vi "_appendClusterFlattenedData.vi"(8 "error in (no error)":errorcluster, 10 "Variant Data":variant, 11 "Flattened Cluster":string) -> (0 "error out":errorcluster, 3 "Appended Cluster":string)   [LabVIEW 2013, in "BSON.lvlib" / "tBSONDocument.lvclass"]
uses:
  tBSONDocument.lvclass
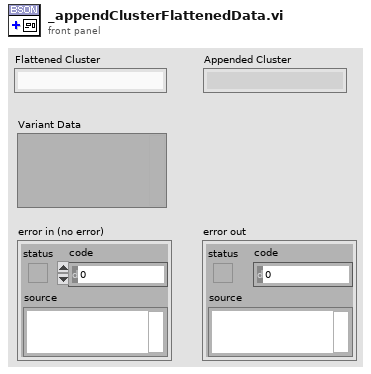
[diagram p1: front panel]
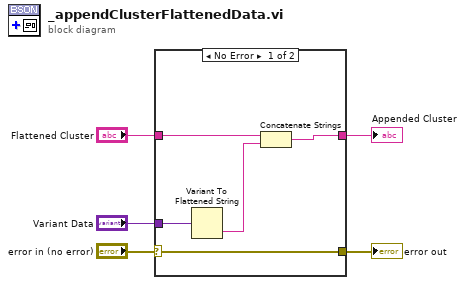
[diagram p0: block diagram]
diagram:
  n1 = case shown="No Error" "error in (no error)" {
    selector: "error in (no error)" -> [w7 w12]
    tunnel: [w7 w12] -> w5
    tunnel: "Flattened Cluster" -> [w9 w11]
    tunnel: "Variant Data" -> [w10 _]
    tunnel: [w6 w11] -> w1
    frame No Error {
      n2 = Variant To Flattened String(Variant=w10) -> (data string=w8:string)  [unwired: 1 out]
      n3 = Concatenate Strings(w9, w8) -> (w6:string)
    }
    frame Error {
    }
  }
  "error out" <- w5
  "Appended Cluster" <- w1
